vi "Initialize.vi"(8 "error in (no error)":errorcluster, 9 "Device":string, 10 "VISA Com Port":refnum<visa-resource-name>, 11 "object in":refnum<class "Cypress.lvclass">) -> (0 "error out":errorcluster, 3 "object out":refnum<class "Cypress.lvclass">)   [LabVIEW 2020, in "Cypress.lvclass"]
doc: "En este vi de inicialización, donde se prepara para abrir la comuniacón entre el software y el micrcontrolado, se ajusta el puerto serial"
uses:
  Cypress.lvclass
  Cypress.lvclass/Cypress.ctl
  <vilib>/Instr/_visa.llb/VISA Configure Serial Port (Instr).vi
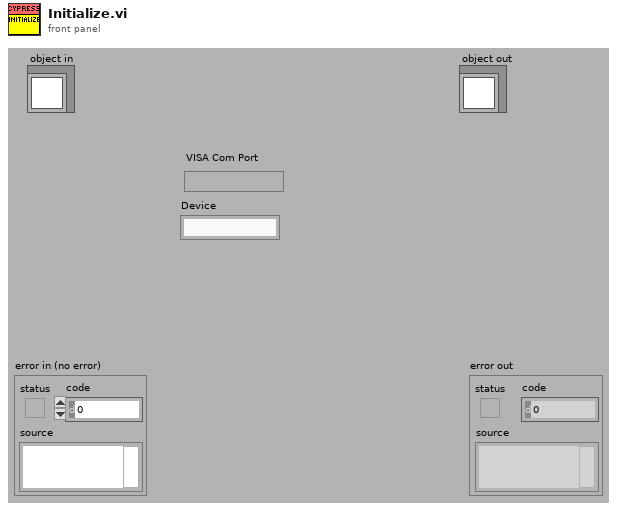
[diagram p1: front panel]
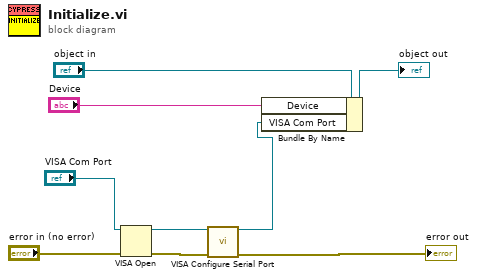
[diagram p0: block diagram]
diagram:
  n1 = VISA Open(error in (no error)="error in (no error)", VISA resource name="VISA Com Port") -> (VISA resource name=w2:refnum<visa-resource-name>, error out=w5:errorcluster)  [unwired: 3 in]
  n2 = call-poly "VISA Configure Serial Port"("VISA resource name"=w2, "error in (no error)"=w5) -> ("VISA resource name out"=w1:refnum<visa-resource-name>, "error out"=→"error out":errorcluster)  [unwired: 12 in]
  n3 = Bundle By Name(cluster="object in", "Device"="Device", "VISA Com Port"=w1) -> (→"object out":refnum<class "Cypress.lvclass">)
